vi "Get Statistics.vi"(8 "error in (no error)":errorcluster, 11 "Result Model in":refnum<class "Result Model.lvclass">) -> (0 "error out":errorcluster, 2 "Results":T1)   [LabVIEW 2020, in "Result Model.lvclass"]
uses:
  Result Model.lvclass
  Statistics.ctl
  Result Model.lvclass/Result Model.ctl
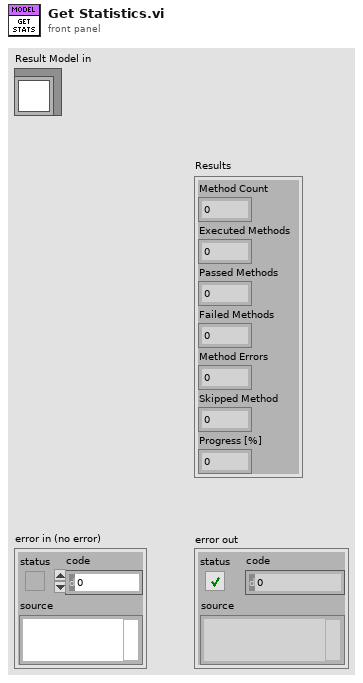
[diagram p1: front panel]
types:
  T1 = typedef "Result Model.lvclass/Statistics.ctl" = cluster{"Method Count":u32, "Executed Methods":u32, "Passed Methods":u32, "Failed Methods":u32, "Method Errors":u32, "Skipped Method":u32, "Progress [%]":dbl}
  T2 = typedef "Result.lvlib/Status.ctl" = enum16{"", "Passed", "Failed", "Error", "Skipped", "Setup Error", "Broken", "Teardown Error"}
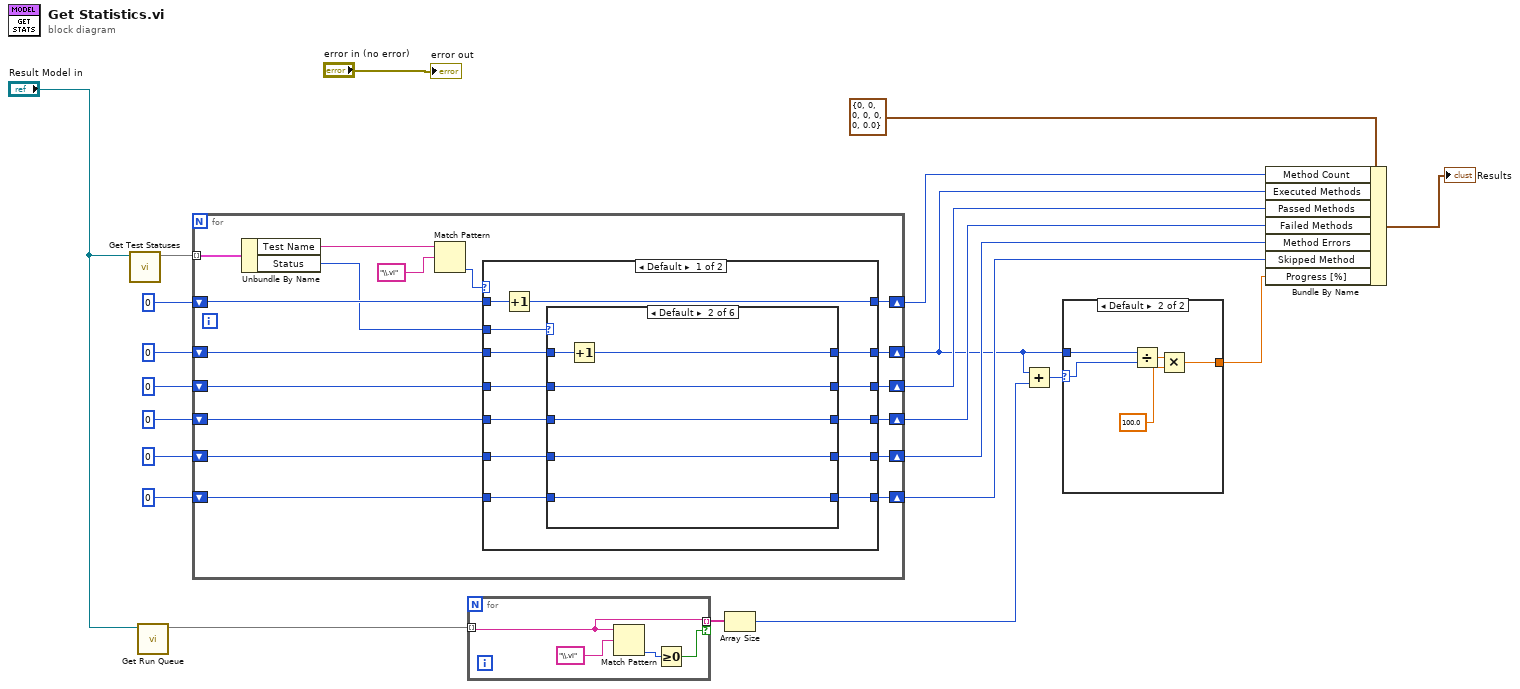
[diagram p0: block diagram]
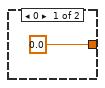
[diagram p2: hidden frame]
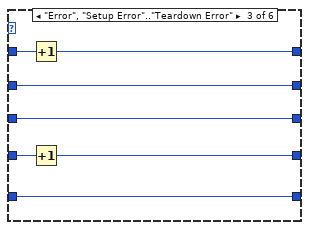
[diagram p4: hidden frame]
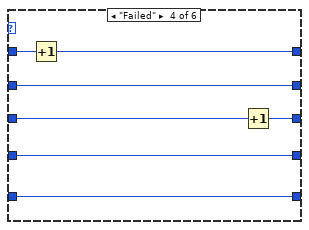
[diagram p5: hidden frame]
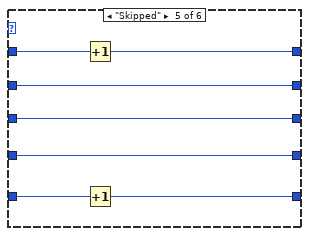
[diagram p6: hidden frame]
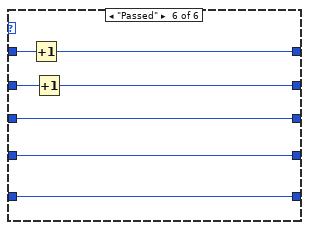
[diagram p7: hidden frame]
diagram:
  n1 = call "Get Test Statuses.vi"("Result Model in"="Result Model in") -> ("Test Statuses"=w4:map{string, T2})  [unwired: 10 in]
  n2 = call "Get Run Queue.vi"("Result Model in"="Result Model in") -> ("Run Queue"=w2:set{string})  [unwired: 10 in]
  n3 = for {
    tunnel: w4 -> [w39] mode=indexing
    shift-right: [w34] -> w10
    shift-left: u32 0 ("Method Count") -> [w35]
    shift-right: [w31] -> w8
    shift-left: u32 0 ("Method Count") -> [w32]
    shift-right: [w29] -> w18
    shift-left: u32 0 ("Method Count") -> [w30]
    shift-right: [w27] -> w16
    shift-left: u32 0 ("Method Count") -> [w28]
    shift-right: [w25] -> w14
    shift-left: u32 0 ("Method Count") -> [w26]
    shift-right: [w23] -> w12
    shift-left: u32 0 ("Method Count") -> [w24]
    n4 = Unbundle By Name(w39) -> ("Test Name"=w38:string, "Status"=w33:T2)
    n5 = Match Pattern(string=w38, regular expression="\\.vi") -> (offset past match=w36:i32)  [unwired: 1 in, 3 out]
    n6 = case shown="Default" w36 {
      tunnel: w35 -> [w52 w97]
      tunnel: [w51 w97] -> w34
      tunnel: w33 -> [w50 _]
      tunnel: w32 -> [w49 w96]
      tunnel: [w48 w96] -> w31
      tunnel: w30 -> [w47 w95]
      tunnel: [w46 w95] -> w29
      tunnel: w28 -> [w45 w94]
      tunnel: [w44 w94] -> w27
      tunnel: w26 -> [w43 w93]
      tunnel: [w42 w93] -> w25
      tunnel: w24 -> [w41 w92]
      tunnel: [w40 w92] -> w23
      frame Default {
        n7 = Increment(x=w52) -> (x+1=w51:u32)
        n8 = case shown="Default" w50 {
          tunnel: w49 -> [w57 w63 w70 w77 w84 w91]
          tunnel: [w57 w62 w69 w76 w83 w90] -> w48
          tunnel: w47 -> [w56 w61 w68 w75 w82 w89]
          tunnel: [w56 w61 w68 w75 w82 w88] -> w46
          tunnel: w45 -> [w55 w60 w67 w74 w81 w87]
          tunnel: [w55 w60 w67 w73 w81 w87] -> w44
          tunnel: w43 -> [w54 w59 w66 w72 w80 w86]
          tunnel: [w54 w59 w65 w72 w80 w86] -> w42
          tunnel: w41 -> [w53 w58 w64 w71 w79 w85]
          tunnel: [w53 w58 w64 w71 w78 w85] -> w40
          frame "" {
          }
          frame Default {
            n9 = Increment(x=w63) -> (x+1=w62:u32)
          }
          frame "Error", "Setup Error".."Teardown Error" {
            n10 = Increment(x=w70) -> (x+1=w69:u32)
            n11 = Increment(x=w66) -> (x+1=w65:u32)
          }
          frame "Failed" {
            n12 = Increment(x=w77) -> (x+1=w76:u32)
            n13 = Increment(x=w74) -> (x+1=w73:u32)
          }
          frame "Skipped" {
            n14 = Increment(x=w84) -> (x+1=w83:u32)
            n15 = Increment(x=w79) -> (x+1=w78:u32)
          }
          frame "Passed" {
            n16 = Increment(x=w91) -> (x+1=w90:u32)
            n17 = Increment(x=w89) -> (x+1=w88:u32)
          }
        }
      }
      frame -1 {
      }
    }
  }
  n18 = for {
    tunnel: w2 -> [w99] mode=indexing
    tunnel: [w99] -> w6 mode=indexing if=w98
    n19 = Match Pattern(string=w99, regular expression="\\.vi") -> (offset past match=w100:i32)  [unwired: 1 in, 3 out]
    n20 = Greater Or Equal To 0?(x=w100) -> (x >= 0?=w98:bool)
  }
  n21 = Array Size(array=w6) -> (size(s)=w5:i32)
  n22 = Add(x=w8, y=w5) -> (x+y=w7:u32)
  n23 = case shown="Default" w7 {
    selector: w7 -> [_ w103]
    tunnel: w8 -> [_ w104]
    tunnel: [0.0 w105] -> w9
    frame 0 {
    }
    frame Default {
      n24 = Divide(x=w104, y=w103) -> (x/y=w107:dbl)
      n25 = Multiply(x=w107, y=100.0) -> (x*y=w105:dbl)
    }
  }
  n26 = Bundle By Name(cluster=T1 {"Method Count"=0, "Executed Methods"=0, "Passed Methods"=0, "Failed Methods"=0, "Method Errors"=0, "Skipped Method"=0, "Progress [%]"=0.0} ("Results"), "Method Count"=w10, "Executed Methods"=w8, "Passed Methods"=w18, "Failed Methods"=w16, "Method Errors"=w14, "Skipped Method"=w12, "Progress [%]"=w9) -> (→"Results":T1)
  "error out" <- "error in (no error)"
